vi "Query AM Properties.vi"(0 "VISA resource name":refnum<visa-resource-name>, 5 "Channel (0: Channel 1)":T1 items=["Channel 1", "Channel 2"], 11 "error in (no error)":errorcluster) -> (4 "VISA resource name out":refnum<visa-resource-name>, 6 "AM Source":u16(ring) items=["Internal", "External"], 8 "Modulation Waveform":u16(ring) items=["Sine", "Square", "Triangle", "Ramp", "Down Ramp", "Noise"], 10 "Modulation Frequency":dbl[unit]=1000.0, 14 "Modulation Depth":dbl, 15 "error out":errorcluster)   [LabVIEW 2023, in "Tektronix AFG 3000 Series.lvlib"]
uses:
  Tektronix AFG 3000 Series.lvlib
  controls.llb/Channel.ctl
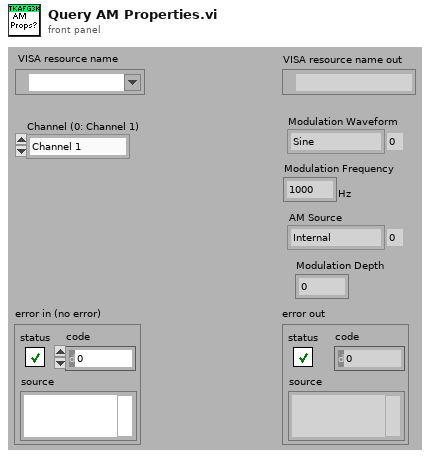
[diagram p1: front panel]
types:
  T1 = typedef "Channel.ctl" = u16
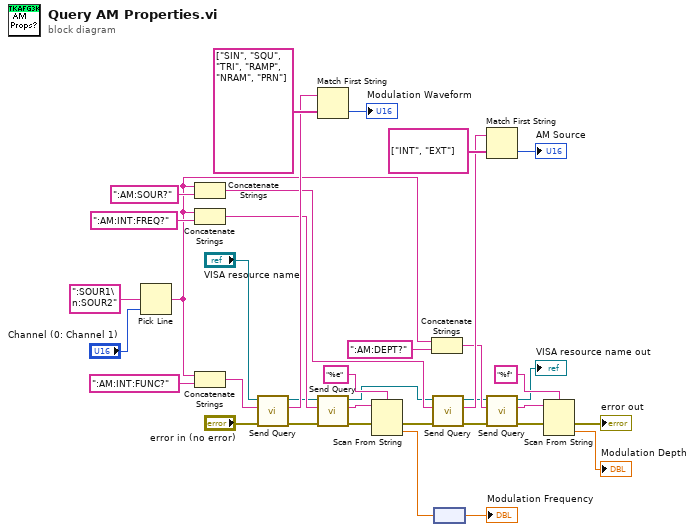
[diagram p0: block diagram]
diagram:
  n1 = Pick Line(multi-line string=":SOUR1\n:SOUR2" ("string (\"\")"), line index="Channel (0: Channel 1)") -> (output string=w10:string)  [unwired: 1 out]
  n2 = Concatenate Strings(w10, ":AM:SOUR?" ("string")) -> (w20:string)
  n3 = Concatenate Strings(w10, ":AM:INT:FREQ?" ("string")) -> (w28:string)
  n4 = Concatenate Strings(w10, ":AM:INT:FUNC?" ("string")) -> (w32:string)
  n5 = call "Send Query.vi"("error in (no error)"="error in (no error)", "write buffer"=w32, "VISA resource name"="VISA resource name") -> ("error out"=w23:errorcluster, "read buffer"=w31:string, "VISA resource name out"=w22:refnum<visa-resource-name>)  [unwired: 1 in, 5 out]
  n6 = Match First String(2:string[] ["SIN", "SQU", "TRI", "RAMP", "NRAM", "PRN"], 3:w31) -> (0:→"Modulation Waveform":i32)  [unwired: 1 out]
  n7 = call "Send Query.vi"("error in (no error)"=w23, "write buffer"=w28, "VISA resource name"=w22) -> ("error out"=w15:errorcluster, "read buffer"=w26:string, "VISA resource name out"=w4:refnum<visa-resource-name>)  [unwired: 1 in, 5 out]
  n8 = Scan From String(format string="%e", input string=w26, error in=w15) -> (error out=w14:errorcluster, output 1=w25:dbl)  [unwired: 1 in, 3 out]
  n9 = Concatenate Strings(w10, ":AM:DEPT?" ("string")) -> (w11:string)
  n10 = call "Send Query.vi"("error in (no error)"=w14, "write buffer"=w20, "VISA resource name"=w4) -> ("error out"=w13:errorcluster, "read buffer"=w18:string, "VISA resource name out"=w3:refnum<visa-resource-name>)  [unwired: 1 in, 5 out]
  n11 = node(w25) -> (→"Modulation Frequency":dbl[unit])
  n12 = Match First String(2:string[] ["INT", "EXT"], 3:w18) -> (0:→"AM Source":i32)  [unwired: 1 out]
  n13 = call "Send Query.vi"("error in (no error)"=w13, "write buffer"=w11, "VISA resource name"=w3) -> ("error out"=w8:errorcluster, "read buffer"=w7:string, "VISA resource name out"=→"VISA resource name out":refnum<visa-resource-name>)  [unwired: 1 in, 5 out]
  n14 = Scan From String(format string="%f", input string=w7, error in=w8) -> (error out=→"error out":errorcluster, output 1=→"Modulation Depth":dbl)  [unwired: 2 in, 2 out]
